vi "Ref. Gen.vi"(7 "Signal Cluster":T1={"phase"=0.0, "amplitude"=1.0, "frequency"=0.3, "offset"=1.0, "Signal"=enum."Sine"} {"offset" format="%0.2f"; "frequency" format="%0.2f"; "amplitude" format="%0.2f"; "phase" format="%0.2f"}, 9 "AI Ref. cmd":dbl, 10 "Ref. cmd.":dbl(slide) step=1.0 scale=-10.0..10.0 scale format="%#.1f", 11 "Ref. Gen.":enum32{"Analog In", "Manual", "Wave Gen"}(tab)=enum."Manual") -> ()   [LabVIEW 2016]
doc: "Signal Reference Subsystem\nType of reference and ref. command as input. - generates ref. value as output."
uses:
  <vilib>/Simulation/Implementation/Shared/SIMSCR Execution Mode.ctl
  <vilib>/Simulation/Scripting/Companion Diagram/SimConfigNode/SimParams.ctl
  <vilib>/Simulation/Scripting/Companion Diagram/SimConfigNode/_simSolvers.ctl
  <vilib>/Simulation/Param Hierarchy/Typedefs/SIMPH Param Control Actions.ctl
  <vilib>/Simulation/Implementation/Shared/NILVSim_ParamChanged.vi
  <vilib>/Simulation/Implementation/Shared/NILVSIM_BeginStep.vi
  <vilib>/Simulation/Implementation/Shared/SIM Is Init or Final Stage.vi
  <vilib>/Simulation/DataSources/Implementation/NILVSim Signal Generator.llb/SIM Signal Generator (scalar).vi
  <vilib>/Simulation/Implementation/Shared/NILVSim_Manager.vi
  <vilib>/Utility/error.llb/Clear Errors.vi
  <vilib>/Simulation/Implementation/Shared/NILVSim_FinalizeModel.vi
  <vilib>/Simulation/Implementation/Shared/SIM Unbundle Sim Info.vi
  <vilib>/Simulation/Implementation/Shared/SIMSH Read Queue.vi
  <vilib>/Simulation/Implementation/Shared/NILVSim_Initialize.vi
  <vilib>/Simulation/Utility/Implementation/NILVSim Get Time and IsAcceptedStep.vi
  <vilib>/Simulation/Implementation/Shared/NILVSim_GetModelError.vi
  <vilib>/Simulation/Implementation/Shared/SIM SimErrorHandler.vi
  <vilib>/Simulation/Implementation/Shared/SIM Bundle Sim Info.vi
  <vilib>/Simulation/Scripting/Companion Diagram/SimConfigNode/SimDog.xnode
  <vilib>/Simulation/Implementation/XNodeFramework/SimXNode/SimX.xnode
  <vilib>/Simulation/Implementation/Shared/NI_SIM_Implementation.lvlib
panel:
  out "Ref. Value":dbl
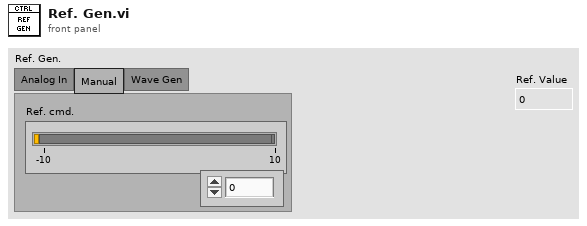
[diagram p1: front panel]
types:
  T1 = cluster{"phase":dbl, "amplitude":dbl, "frequency":dbl, "offset":dbl, "Signal":enum16{"Sine", "Square", "Sawtooth", "Random"}}
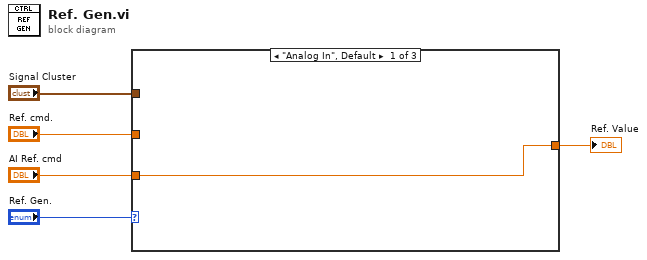
[diagram p0: block diagram]
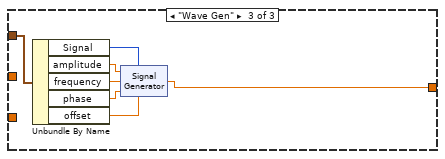
[diagram p3: hidden frame]
diagram:
  n1 = case shown="\"Analog In\", Default" "Ref. Gen." {
    tunnel: "Signal Cluster" -> [_ _ w14]
    tunnel: [w6 w7 w13] -> w2
    tunnel: "Ref. cmd." -> [_ w7 _]
    tunnel: "AI Ref. cmd" -> [w6 _ _]
    frame "Analog In", Default {
    }
    frame "Manual" {
    }
    frame "Wave Gen" {
      n2 = Unbundle By Name ("Unbundle By Name 2")(w14) -> ("Signal"=w12:enum16{"Sine", "Square", "Sawtooth", "Random"}, "amplitude"=w11:dbl, "frequency"=w10:dbl, "phase"=w9:dbl, "offset"=w8:dbl)
      n3 = xnode "Signal Generator"("amplitude"=w11, "signal type"=w12, "frequency"=w10, "phase"=w9, "offset"=w8) -> ("output"=w13:dbl)  [unwired: 2 in]
    }
  }
  "Ref. Value" <- w2
